vi "DHE.vi"(0 "modpath":path, 7 "Cmd":string, 11 "error in":errorcluster) -> (4 "ImmedReplyString":string, 6 "DHE_DBSRef":T1, 10 "TimeOut out":i32, 15 "error out":errorcluster)   [LabVIEW 2016]
uses:
  DBSHAND/private/vis/DatabaseHand_RefNum.ctl
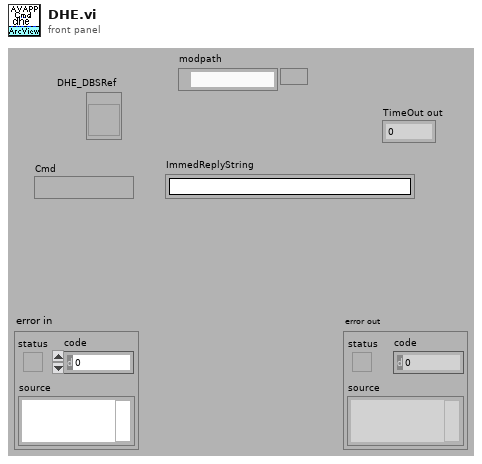
[diagram p1: front panel]
types:
  T1 = typedef "DatabaseHand_RefNum.ctl" = refnum<vi>
  T2 = typedef "DHE_Device.ctl" = cluster{"DevNo":i32, "fd":i32, "name":string, "FPA":string, "modifiers":string, "binpatt":string, "readtime":dbl, "readmode":string, "type":string, "params":string}
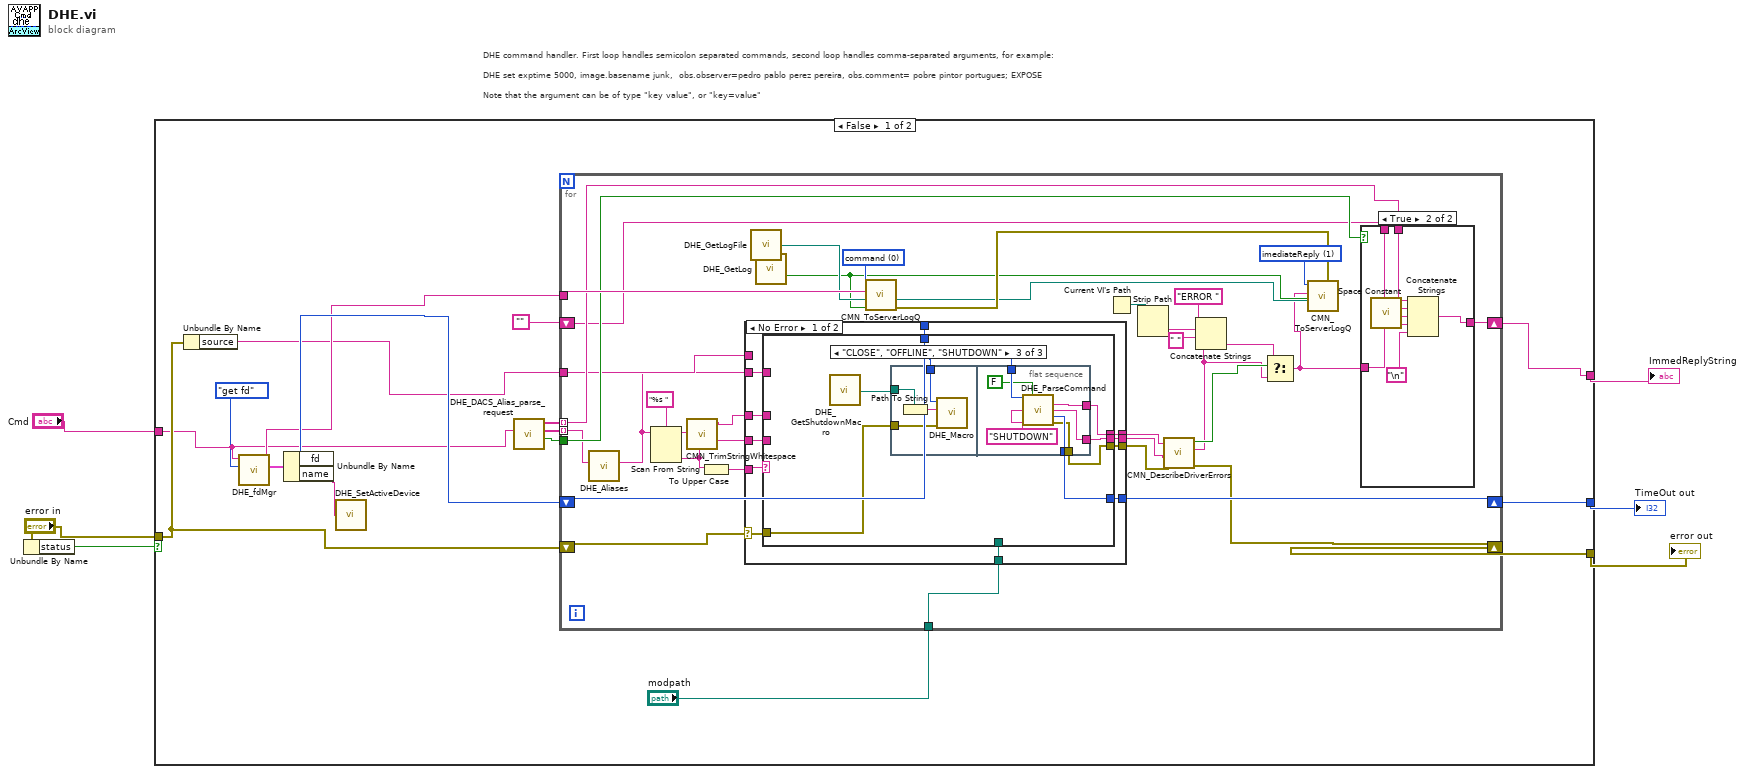
[diagram p0: block diagram]
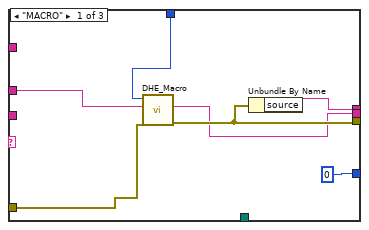
[diagram p3: hidden frame]
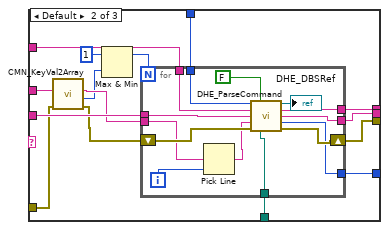
[diagram p4: hidden frame]
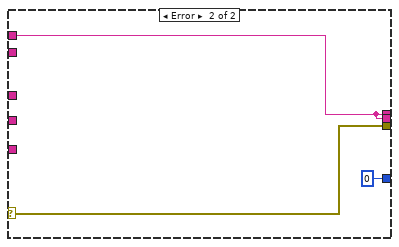
[diagram p5: hidden frame]
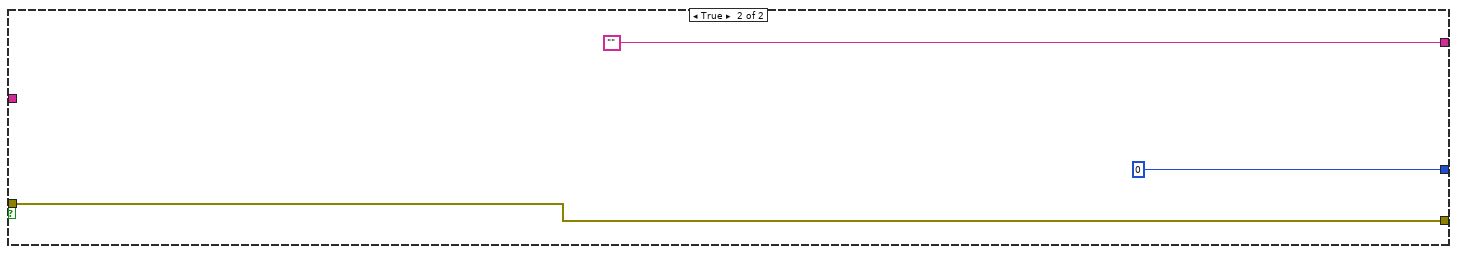
[diagram p6: hidden frame]
diagram:
  # "DHE command handler. First loop handles semicolon separated commands, second loop handles comma-separated arguments, for example:\n\nDHE set exptime 5000, image.basename junk,  obs.observer=pedro pablo perez pereira, obs.comment= pobre pintor portugues; EXPOSE\n\nNote that the argument can be of type \"key value\", or \"key=value\""
  n1 = Unbundle By Name("error in") -> ("status"=w3:bool)
  n2 = case shown="False" w3 {
    tunnel: "error in" -> [w15 w134]
    tunnel: [w16 w134] -> w6
    tunnel: [w12 ""] -> w5
    tunnel: "Cmd" -> [w7 _]
    tunnel: [w18 0 ("TimeOut out")] -> w1
    frame False {
      n3 = Unbundle By Name(w15) -> ("source"=w13:string)
      n4 = call "DHE_fdMgr.vi"("action"=enum16{"get fd", "set fd"}."get fd", "cmd in"=w7) -> ("Device"=w21:T2, "cmd out"=w17:string)  [unwired: 3 in, 5 out]
      n5 = Unbundle By Name(w21) -> ("fd"=w20:i32, "name"=w19:string)
      n6 = call "DHE_SetActiveDevice.vi"("DHE_ActiveDevice"=w19) -> ()  [unwired: 9 out]
      n7 = call "DHE_DACS_Alias_parse_request.vi"("cmd in"=w7) -> ("mult. aliases?"=w10:bool, "cmds out"=w11:string[], "alias names"=w9:string[])  [unwired: 7 in, 1 out]
      n8 = for {
        tunnel: w17 -> [w54]
        tunnel: "modpath" -> [w50]
        shift-right: [w55] -> w18
        shift-left: w20 -> [w56]
        shift-right: [w53] -> w16
        shift-left: w15 -> [w52]
        tunnel: w11 -> [w24] mode=indexing
        tunnel: w10 -> [w30]
        tunnel: w9 -> [w28] mode=indexing
        shift-right: [w27] -> w12
        shift-left: "" -> [w26]
        tunnel: w13 -> [w25]
        w39 = u16 1 items=["command", "imediateReply", "Callback Reply", "Information"] ("type")
        w40 = u16 0 items=["command", "imediateReply", "Callback Reply", "Information"] ("type")
        n9 = call "DHE_Aliases.vi"("name in"=w24) -> ("name out"=w23:string)  [unwired: 7 in, 3 out]
        n10 = Scan From String(format string="%s " ("Format String"), input string=w23) -> (remaining string=w34:string, output 1=w33:string)  [unwired: 2 in, 3 out]
        n11 = call "CMN_TrimStringWhitespace.vi"("string"=w34) -> ("trimmed string"=w31:string)  [unwired: 1 in, 8 out]
        n12 = To Upper Case(1:w33) -> (0:w32:string)
        n13 = case shown="No Error" w52 {
          selector: w52 -> [w65 w131]
          tunnel: [w74 w129] -> w51
          tunnel: [w73 w131] -> w42
          tunnel: [w72 w129] -> w41
          tunnel: w56 -> [w71 _]
          tunnel: [w70 0 ("TimeOut out")] -> w55
          tunnel: w33 -> [w69 _]
          tunnel: w32 -> [w68 _]
          tunnel: w31 -> [w67 _]
          tunnel: w23 -> [w66 _]
          tunnel: w25 -> [_ w129]
          tunnel: w50 -> [w64 _]
          frame No Error {
            n14 = case shown="\"CLOSE\", \"OFFLINE\", \"SHUTDOWN\"" w68 {
              tunnel: w66 -> [_ w96 _]
              tunnel: w69 -> [_ w95 _]
              tunnel: [w79 w94 w114] -> w74
              tunnel: w67 -> [w77 w93 _]
              tunnel: w65 -> [w81 w92 w117]
              tunnel: [w80 w89 w111] -> w73
              tunnel: [w76 w86 w112] -> w72
              tunnel: w71 -> [w78 w84 w115]
              tunnel: [0 ("TimeOut out") w83 w113] -> w70
              tunnel: w64 -> [_ w82 _]
              frame "MACRO" {
                n15 = call "DHE_Macro.vi"("error in (no error)"=w81, "macro"=w77, "fd"=w78) -> ("error out"=w80:errorcluster, "response"=w76:string)  [unwired: 1 in, 6 out]
                n16 = Unbundle By Name(w80) -> ("source"=w79:string)
              }
              frame Default {
                n17 = call "CMN_KeyVal2Array.vi"("error in (no error)"=w92, "command in"=w93) -> ("error out"=w90:errorcluster, "number of commands"=w88:i32, "commands out"=w91:string)  [unwired: 1 in, 5 out]
                n18 = Max & Min(x=1, y=w88) -> (max(x,y)=w85:i32)  [unwired: 1 out]
                n19 = for {
                  N: w85 -> [_]
                  tunnel: w84 -> [w110]
                  tunnel: w96 -> [w109]
                  tunnel: w95 -> [w108]
                  tunnel: [w107] -> w94
                  tunnel: w91 -> [w103]
                  shift-right: [w105] -> w89
                  shift-left: w90 -> [w106]
                  tunnel: [w101] -> w86
                  tunnel: [w100] -> w83
                  tunnel: w82 -> [w98]
                  i -> [w104]
                  n20 = Pick Line(multi-line string=w103, line index=w104) -> (output string=w102:string)  [unwired: 1 out]
                  n21 = call "DHE_ParseCommand.vi"("fd"=w110, "Log"=FALSE, "command + args"=w109, "command"=w108, "arguments"=w102, "error in"=w106, "modpath"=w98) -> ("DHE_DBSRef"=→"DHE_DBSRef":T1, "message"=w107:string, "OK message"=w101:string, "TimeOut out"=w100:i32, "error out"=w105:errorcluster)  [unwired: 4 out]
                }
              }
              frame "CLOSE", "OFFLINE", "SHUTDOWN" {
                n22 = call "DHE_GetShutdownMacro.vi"() -> ("DHE_InitMacro"=w116:path)  [unwired: 9 out]
                n23 = flat-sequence {
                  tunnel: w117 -> [w121]
                  tunnel: w115 -> [w120]
                  tunnel: w116 -> [w119]
                  tunnel: w115 -> [w128]
                  tunnel: [w126] -> w114
                  tunnel: [w125] -> w113
                  tunnel: [w124] -> w112
                  tunnel: [w123] -> w111
                  frame #0 {
                    n24 = Path To String(path=w119) -> (string=w118:string)
                    n25 = call "DHE_Macro.vi"("error in (no error)"=w121, "macro"=w118, "fd"=w120) -> ()  [unwired: 1 in, 8 out]
                  }
                  frame #1 {
                    n26 = call "DHE_ParseCommand.vi"("fd"=w128, "Log"=FALSE, "command"="SHUTDOWN") -> ("message"=w126:string, "OK message"=w124:string, "TimeOut out"=w125:i32, "error out"=w123:errorcluster)  [unwired: 4 in, 5 out]
                  }
                }
              }
            }
          }
          frame Error {
          }
        }
        n27 = call "DHE_GetLogFile.vi"() -> ("DHE_LogFile"=w37:path)  [unwired: 9 out]
        n28 = call "DHE_GetLog.vi"() -> ("DHE_log"=w36:bool)  [unwired: 9 out]
        n29 = call "CMN_ToServerLogQ.vi"("Log"=w36, "file"=w37, "string"=w54, "type"=w40) -> ("error out"=w38:errorcluster)  [unwired: 2 in, 4 out]
        n30 = Current VI's Path() -> (path=w47:path)
        n31 = Strip Path(path=w47) -> (name=w46:string)  [unwired: 1 out]
        n32 = call "CMN_DescribeDriverErrors.vi"("message"=w51, "OK message"=w41, "error in (no error)"=w42) -> ("error?"=w44:bool, "astroerrors"=w43:string, "error out"=w53:errorcluster)  [unwired: 1 in, 4 out]
        n33 = Concatenate Strings("ERROR ", w46, " ", w43) -> (w48:string)
        n34 = Select(t=w48, s=w44, f=w43) -> (s? t:f=w29:string)
        n35 = call "CMN_ToServerLogQ.vi"("error in (no error)"=w38, "Log"=w36, "file"=w37, "string"=w29, "type"=w39) -> ()  [unwired: 1 in, 5 out]
        n36 = case shown="True" w30 {
          tunnel: w29 -> [w57 w63]
          tunnel: [w57 w58] -> w27
          tunnel: w28 -> [_ w60]
          tunnel: w26 -> [_ w59]
          frame False {
          }
          frame True {
            n37 = call <vilib>:"Space Constant.vi"() -> ("String"=w62:string)
            n38 = Concatenate Strings(w59, w60, w62, w63, "\n") -> (w58:string)
          }
        }
      }
    }
    frame True {
    }
  }
  "error out" <- w6
  "ImmedReplyString" <- w5
  "TimeOut out" <- w1
